vi "Example Output.vi"() -> ()   [LabVIEW 2010]
uses:
  C:/tf/play/labview/Tinkerforge.dll
panel:
  in  "uid":string="aE7"
  in  "port":i32=4223
  in  "host":string="localhost"
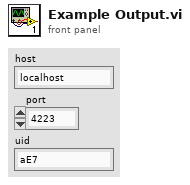
[diagram p1: front panel]
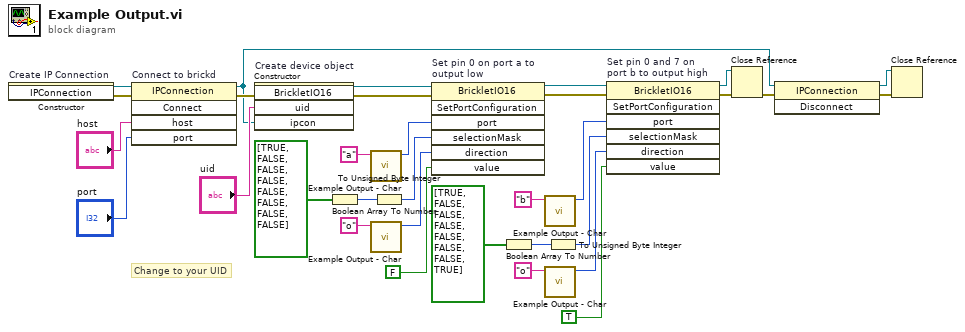
[diagram p0: block diagram]
diagram:
  # "Change to your UID"
  n1 = constructor on="Create IP Connection" class="IPConnection"() -> (reference out=w32:refnum<k24>, error out=w21:errorcluster)  [unwired: 3 in, 1 out]
  n2 = invoke on="Connect to brickd" class="IPConnection" method="Connect"(reference=w32, error in=w21, "host"="host", "port"="port") -> (reference out=w23:refnum<k24>, error out=w28:errorcluster)  [unwired: 1 in, 3 out]
  n3 = constructor on="Create device object" class="BrickletIO16"(error in=w28, "uid"="uid", "ipcon"=w23) -> (reference out=w26:refnum<k24>, error out=w27:errorcluster)  [unwired: 2 in, 3 out]
  n4 = Boolean Array To Number(Boolean array=bool[] [TRUE, FALSE, FALSE, FALSE, FALSE, FALSE, FALSE, FALSE]) -> (number=w18:u32)
  n5 = call "Example Output - Char.vi"("string"="a") -> ("char"=w16:u16)  [unwired: 10 in]
  n6 = call "Example Output - Char.vi"("string"="o") -> ("char"=w14:u16)  [unwired: 10 in]
  n7 = To Unsigned Byte Integer(number=w18) -> (unsigned 8bit integer=w19:u8)
  n8 = invoke on="Set pin 0 on port a to\noutput low" class="BrickletIO16" method="SetPortConfiguration"(reference=w26, error in=w27, "port"=w16, "selectionMask"=w19, "direction"=w14, "value"=FALSE) -> (reference out=w11:refnum<k24>, error out=w12:errorcluster)  [unwired: 1 in, 5 out]
  n9 = Boolean Array To Number(Boolean array=bool[] [TRUE, FALSE, FALSE, FALSE, FALSE, FALSE, FALSE, TRUE]) -> (number=w2:u32)
  n10 = call "Example Output - Char.vi"("string"="b") -> ("char"=w6:u16)  [unwired: 10 in]
  n11 = call "Example Output - Char.vi"("string"="o") -> ("char"=w5:u16)  [unwired: 10 in]
  n12 = To Unsigned Byte Integer(number=w2) -> (unsigned 8bit integer=w1:u8)
  n13 = invoke on="Set pin 0 and 7 on\nport b to output high" class="BrickletIO16" method="SetPortConfiguration"(reference=w11, error in=w12, "port"=w6, "selectionMask"=w1, "direction"=w5, "value"=TRUE) -> (reference out=w10:refnum<k24>, error out=w9:errorcluster)  [unwired: 1 in, 5 out]
  n14 = Close Reference(reference=w10, error in (no error)=w9) -> (error out=w25:errorcluster)
  n15 = invoke class="IPConnection" method="Disconnect"(reference=w23, error in=w25) -> (reference out=w22:refnum<k24>, error out=w24:errorcluster)  [unwired: 1 in, 1 out]
  n16 = Close Reference(reference=w22, error in (no error)=w24) -> ()  [unwired: 1 out]
